vi "writeLoopTimeSV.vi"(8 "error in (no error)":errorcluster, 10 "loopTime_ms":dbl, 11 "LoopTimer in":refnum<class "LoopTimer.lvclass">) -> (0 "error out":errorcluster, 3 "LoopTimer out":refnum<class "LoopTimer.lvclass">)   [LabVIEW 2013, in "ComponentData.lvlib" / "LoopTimer.lvclass"]
uses:
  <userlib>/Common/Component/common_application/RT/ComponentData/LoopTimer/LoopTimer.lvclass
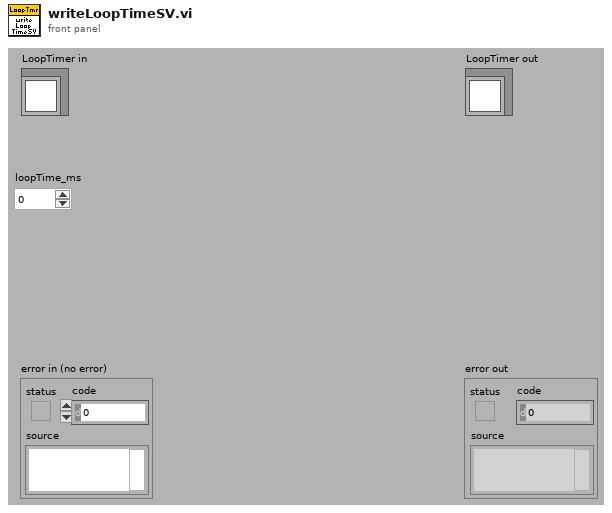
[diagram p1: front panel]
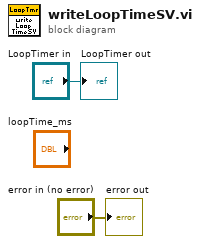
[diagram p0: block diagram]
diagram:
  "error out" <- "error in (no error)"
  "LoopTimer out" <- "LoopTimer in"
